vi "Update.vi"(8 "error in (no error)":errorcluster, 11 "Config Monitor Module in":refnum<class "Config Monitor Module.lvclass">) -> (0 "error out":errorcluster, 3 "Config Monitor Module out":refnum<class "Config Monitor Module.lvclass">, 4 "Node Config Info":T1[](array[typedef]))   [LabVIEW 2020, in "Volatus.lvlib" / "Config Monitor Module.lvclass"]
uses:
  Config Monitor Module.lvclass
  Config Monitor Module.lvclass/Config Monitor Module.ctl
  Module/Module.lvclass
  C:/dev/lv20CE/relink/lv-volatus/Volatus/Module/Module.lvclass
  C:/dev/lv20CE/relink/lv-volatus/Volatus/Config Alert Module/Config Monitor Module.lvclass
  Node Config Info.ctl
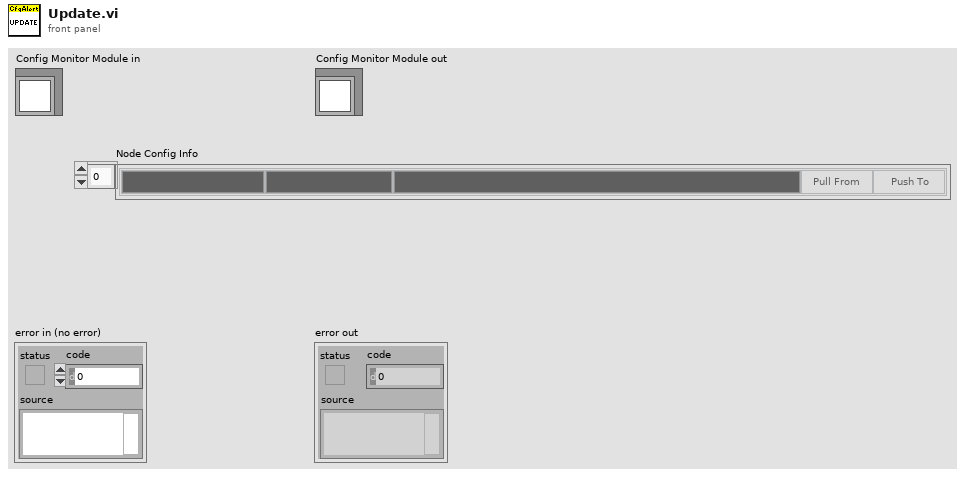
[diagram p1: front panel]
types:
  T1 = typedef "Volatus.lvlib/Config Monitor Module.lvclass/Node Config Info.ctl" = cluster{"Node":string, "Config Version":string, "Config Hash":string, "Pull":bool, "Push":bool, "Version Color":u32, "Hash Color":u32, "Node Color":u32}
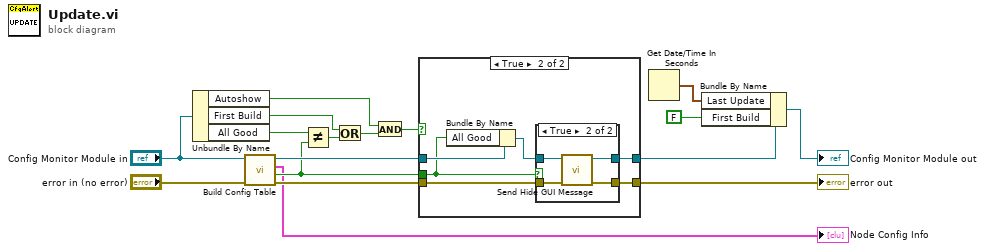
[diagram p0: block diagram]
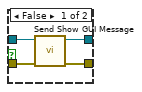
[diagram p3: hidden frame]
diagram:
  n1 = Unbundle By Name("Config Monitor Module in") -> ("Autoshow"=w7:bool, "First Build"=w10:bool, "All Good"=w17:bool)
  n2 = call "Build Config Table.vi"("error in (no error)"="error in (no error)", "Config Alert Module in"="Config Monitor Module in") -> ("error out"=w15:errorcluster, "All Good"=w13:bool, "Node Config Info"=→"Node Config Info":T1[], "Config Alert Module out"=w16:refnum<class "Config Monitor Module.lvclass">)  [unwired: 6 in]
  n3 = Not Equal?(x=w17, y=w13) -> (x != y?=w14:bool)
  n4 = Or(x=w10, y=w14) -> (x .or. y?=w11:bool)
  n5 = And(x=w7, y=w11) -> (x .and. y?=w8:bool)
  n6 = case shown="True" w8 {
    tunnel: w16 -> [w19 w25]
    tunnel: w15 -> [w18 w24]
    tunnel: w13 -> [_ w20]
    tunnel: [w19 w23] -> w12
    tunnel: [w18 w22] -> w3
    frame False {
    }
    frame True {
      n7 = Bundle By Name(cluster=w25, "All Good"=w20) -> (w21:refnum<class "Config Monitor Module.lvclass">)
      n8 = case shown="True" w20 {
        tunnel: w21 -> [w29 w31]
        tunnel: w24 -> [w28 w33]
        tunnel: [w27 w30] -> w23
        tunnel: [w26 w32] -> w22
        frame False {
          n9 = call "Send Show GUI Message.vi"("error in (no error)"=w28, "Module in"=w29) -> ("error out"=w26:errorcluster, "Module out"=w27:refnum<class "Config Monitor Module.lvclass">)  [unwired: 8 in]
        }
        frame True {
          n10 = call "Send Hide GUI Message.vi"("error in (no error)"=w33, "Module in"=w31) -> ("error out"=w32:errorcluster, "Module out"=w30:refnum<class "Config Monitor Module.lvclass">)  [unwired: 8 in]
        }
      }
    }
  }
  "error out" <- w3
  n11 = Get Date/Time In Seconds() -> (seconds since 1Jan1904=w4:timestamp)
  n12 = Bundle By Name(cluster=w12, "Last Update"=w4, "First Build"=FALSE) -> (→"Config Monitor Module out":refnum<class "Config Monitor Module.lvclass">)
